vi "GetActiveFieldName.vi"(1 "protobuf index":i32) -> (0 "oneof field name":string)   [LabVIEW 2019, in "grpc-xnet_client.lvlib" / "nixnet_grpc_ReadStateValue_value.lvclass"]
uses:
  nixnet_grpc_ReadStateValue_value.lvclass
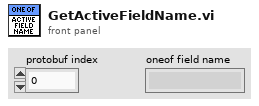
[diagram p1: front panel]
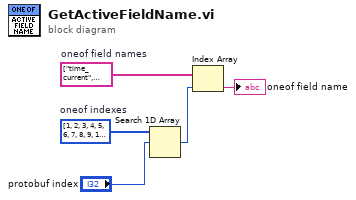
[diagram p0: block diagram]
diagram:
  w5 = string[] ["time_current", "time_communicating", "time_start", "can_comm", "flex_ray_comm", "flex_ray_stats", "lin_comm", "session_info", "j1939_comm_state", "time_current2", "time_communicating2", "time_start2"]  # oneof field names
  w4 = i32[] [1, 2, 3, 4, 5, 6, 7, 8, 9, 10, 11, 12]  # oneof indexes
  n1 = Search 1D Array(1D array=w4, element="protobuf index") -> (index of element=w2:i32)  [unwired: 1 in]
  n2 = Index Array(array=w5, index=w2) -> (element=→"oneof field name":string)
